vi "File_GetAppendedPath.vi"(8 "error in (no error)":errorcluster, 11 "File in":refnum<class "File.lvclass">) -> (0 "error out":errorcluster, 2 "appended path":path, 3 "File out":refnum<class "File.lvclass">)   [LabVIEW 2023, in "File.lvclass"]
uses:
  File.lvclass
  File.lvclass/File.ctl
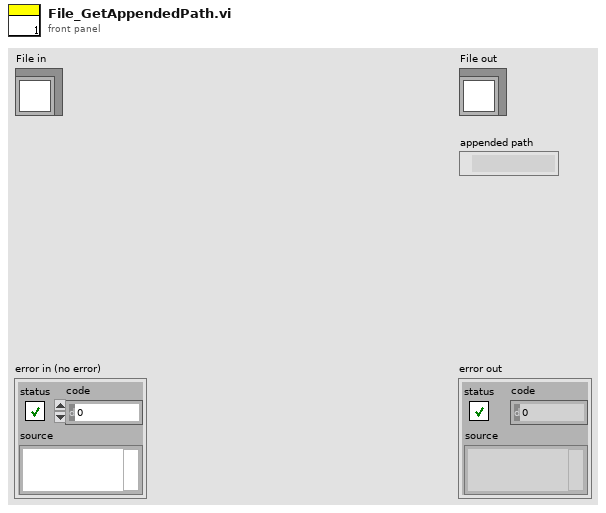
[diagram p1: front panel]
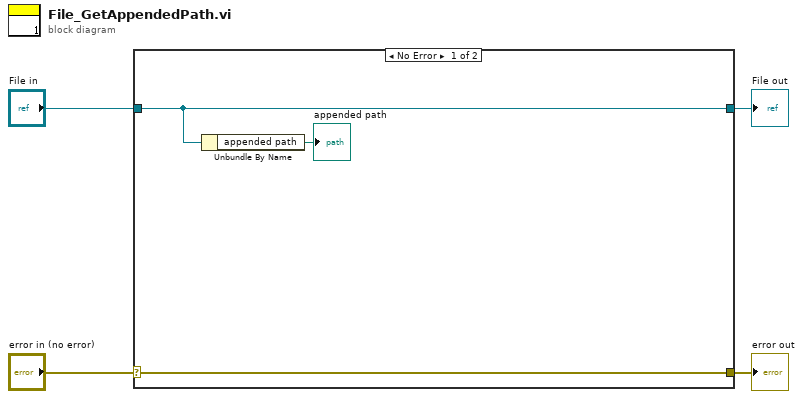
[diagram p0: block diagram]
diagram:
  n1 = case shown="No Error" "error in (no error)" {
    selector: "error in (no error)" -> [w7 w9]
    tunnel: [w7 w9] -> w3
    tunnel: [w6 w8] -> w1
    tunnel: "File in" -> [w6 w8]
    frame No Error {
      n2 = Unbundle By Name(w6) -> ("appended path"=→"appended path":path)
    }
    frame Error {
    }
  }
  "error out" <- w3
  "File out" <- w1
